vi "goal_selecter.vi"(0 "当前索引":i32, 1 "值":T2(array[cluster]), 2 "now_pose_X":dbl, 3 "now_pose_Y":dbl) -> (7 "新索引new":i32, 8 "goal_with_force":T1)   [LabVIEW 2014, in "GlobalPlannerPyPl.lvlib" / "GlobalPlannerPyPl.lvclass"]
uses:
  GlobalPlannerPyPl.lvclass
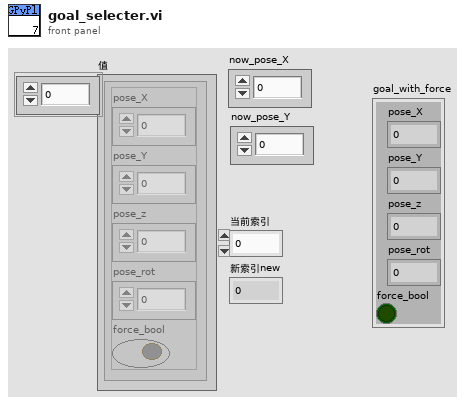
[diagram p1: front panel]
types:
  T1 = cluster{"pose_X":dbl, "pose_Y":dbl, "pose_z":dbl, "pose_rot":dbl, "force_bool":bool}
  T2 = cluster{"pose_X":dbl, "pose_Y":dbl, "pose_z":dbl, "pose_rot":dbl, "force_bool":bool}[]
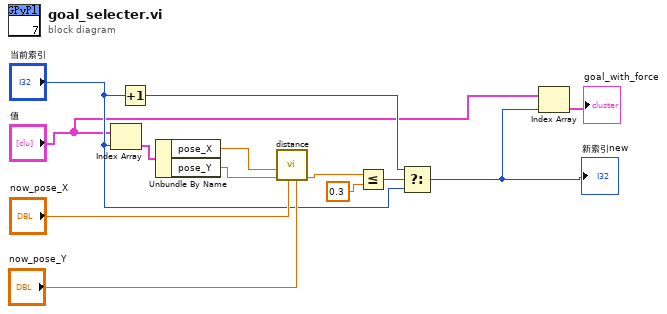
[diagram p0: block diagram]
diagram:
  n1 = Index Array(array="值", index="当前索引") -> (element=w13:T1)
  n2 = Increment(x="当前索引") -> (x+1=w4:i32)
  n3 = Unbundle By Name(w13) -> ("pose_X"=w12:dbl, "pose_Y"=w11:dbl)
  n4 = call "distance.vi"("y2"="now_pose_Y", "x2"="now_pose_X", "y1"=w11, "x1"=w12) -> ("distancex1x2y1y2"=w8:dbl)  [unwired: 6 in, 1 out]
  n5 = Less Or Equal?(x=w8, y=0.3) -> (x <= y?=w6:bool)
  n6 = Select(t=w4, s=w6, f="当前索引") -> (s? t:f=w1:i32)
  "新索引new" <- w1
  n7 = Index Array(array="值", index=w1) -> (element=→"goal_with_force":T1)
